vi "Key Length.vi"(8 "Error In":errorcluster, 11 "Known Host In":refnum<class "KnownHost.lvclass">) -> (0 "Error Out":errorcluster, 2 "Length":u64, 3 "Known Host Out":refnum<class "KnownHost.lvclass">)   [LabVIEW 2017, in "Toolkit.lvlib" / "KnownHost.lvclass"]
uses:
  KnownHost.lvclass
  KnownHost.lvclass/KnownHost.ctl
  Toolkit.lvlib
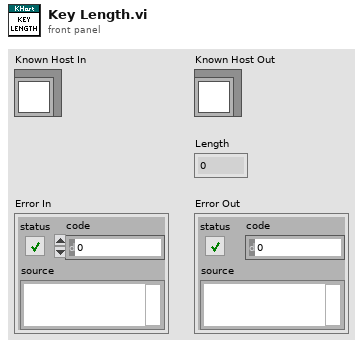
[diagram p1: front panel]
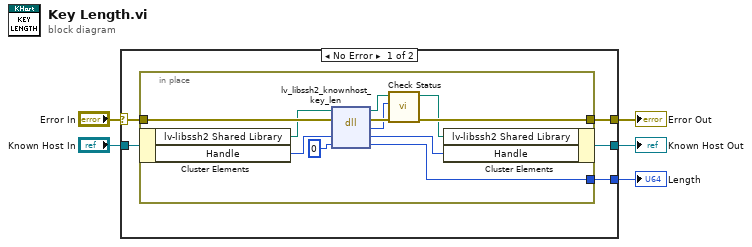
[diagram p0: block diagram]
diagram:
  n1 = case shown="No Error" "Error In" {
    selector: "Error In" -> [w10 w23]
    tunnel: [w9 w23] -> w4
    tunnel: "Known Host In" -> [w8 w22]
    tunnel: [w7 w22] -> w2
    tunnel: [w6 _] -> w1
    frame No Error {
      n2 = in-place {
        in-place-border: w10 -> [w21]
        in-place-border: [w16] -> w9
        in-place-border: [w12] -> w6
        n3 = in-place-cluster #1(w8) -> ("lv-libssh2 Shared Library"=w20:path, "Handle"=w19:u64)
        n4 = dll-call lib="lv-libssh2.*" fn="lv_libssh2_knownhost_key_len"(path in=w20, error in=w21, "handle"=w19, "length"=u64 0) -> (path out=w15:path, error out=w17:errorcluster, "status"=w13:i32, "handle"=w18:u64, "length"=w12:u64)  [unwired: 1 in]
        n5 = call "Check Status.vi"("Error In"=w17, "Status"=w13, "lv-libssh2 Shared Library In"=w15) -> ("Error Out"=w16:errorcluster, "lv-libssh2 Shared Library Out"=w14:path)  [unwired: 7 in]
        n6 = in-place-cluster #1("lv-libssh2 Shared Library"=w14, "Handle"=w18) -> (w7:refnum<class "KnownHost.lvclass">)
      }
    }
    frame Error {
    }
  }
  "Error Out" <- w4
  "Known Host Out" <- w2
  "Length" <- w1
